vi "Joystick control (SubVI).vi"() -> (0 "G+":bool, 1 "M-":bool, 2 "M+":bool, 3 "G-":bool, 4 "Left+":bool, 5 "Right-":bool, 6 "Left-":bool, 7 "Right+":bool)   [LabVIEW 2017]
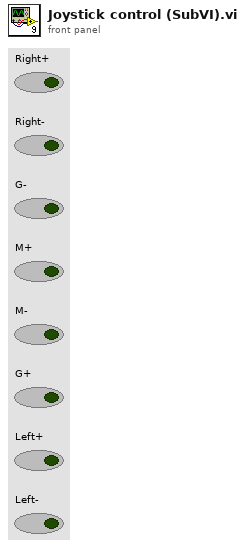
[diagram p1: front panel]
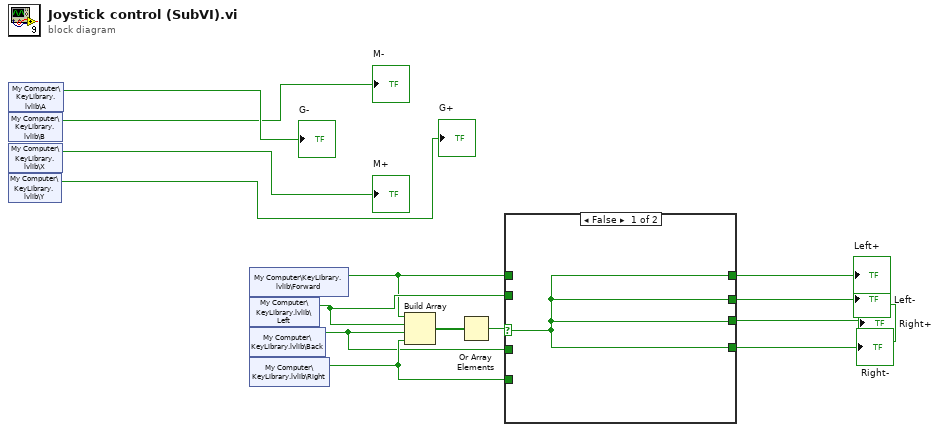
[diagram p0: block diagram]
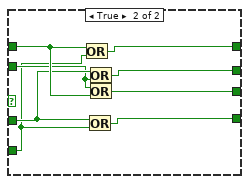
[diagram p2: hidden frame]
diagram:
  n1 = shared-variable "My Computer\\KeyLibrary.lvlib\\A"() -> (→"G-":bool)  [unwired: 1 in, 1 out]
  n2 = shared-variable "My Computer\\KeyLibrary.lvlib\\B"() -> (→"M-":bool)  [unwired: 1 in, 1 out]
  n3 = shared-variable "My Computer\\KeyLibrary.lvlib\\X"() -> (→"M+":bool)  [unwired: 1 in, 1 out]
  n4 = shared-variable "My Computer\\KeyLibrary.lvlib\\Y"() -> (→"G+":bool)  [unwired: 1 in, 1 out]
  n5 = shared-variable "My Computer\\KeyLibrary.lvlib\\Forward"() -> (w7:bool)  [unwired: 1 in, 1 out]
  n6 = shared-variable "My Computer\\KeyLibrary.lvlib\\Left"() -> (w9:bool)  [unwired: 1 in, 1 out]
  n7 = shared-variable "My Computer\\KeyLibrary.lvlib\\Back"() -> (w8:bool)  [unwired: 1 in, 1 out]
  n8 = shared-variable "My Computer\\KeyLibrary.lvlib\\Right"() -> (w10:bool)  [unwired: 1 in, 1 out]
  n9 = Build Array(w7, w9, w8, w10) -> (w6:bool[])
  n10 = Or Array Elements(Boolean array=w6) -> (logical OR=w5:bool)
  n11 = case shown="False" w5 {
    selector: w5 -> [w15 _]
    tunnel: w7 -> [_ w23]
    tunnel: w8 -> [_ w22]
    tunnel: w9 -> [_ w21]
    tunnel: w10 -> [_ w20]
    tunnel: [w15 w19] -> w11
    tunnel: [w15 w18] -> w12
    tunnel: [w15 w17] -> w13
    tunnel: [w15 w16] -> w14
    frame False {
    }
    frame True {
      n12 = Or(x=w23, y=w20) -> (x .or. y?=w17:bool)
      n13 = Or(x=w22, y=w20) -> (x .or. y?=w16:bool)
      n14 = Or(x=w22, y=w21) -> (x .or. y?=w18:bool)
      n15 = Or(x=w21, y=w23) -> (x .or. y?=w19:bool)
    }
  }
  "Right-" <- w14
  "Left+" <- w13
  "Left-" <- w12
  "Right+" <- w11
